vi "Set Waveform.vi"(7 "Treatment of Infinity/NaN":T1, 8 "error in (no error)":errorcluster, 10 "waveform":waveform(dbl), 11 "JSON Object in":refnum<class "JSON Object.lvclass">) -> (0 "error out":errorcluster, 3 "JSON Object out":refnum<class "JSON Object.lvclass">)   [LabVIEW 2020, in "Library Commun.lvlib" / "JSON Object.lvclass"]
uses:
  JSON Object.lvclass
  C:/Users/ngarcin/OneDrive - Altyor/Standard TB/Class/JSON API/JSON Value/JSON Value.lvclass
  JSON Scalar/Infinity&NaN.ctl
  JSON Array/JSON Array.lvclass
  JSON Scalar/JSON Scalar.lvclass
  Variant JSON/Variant JSON.lvlib
  support/JSON support.lvlib
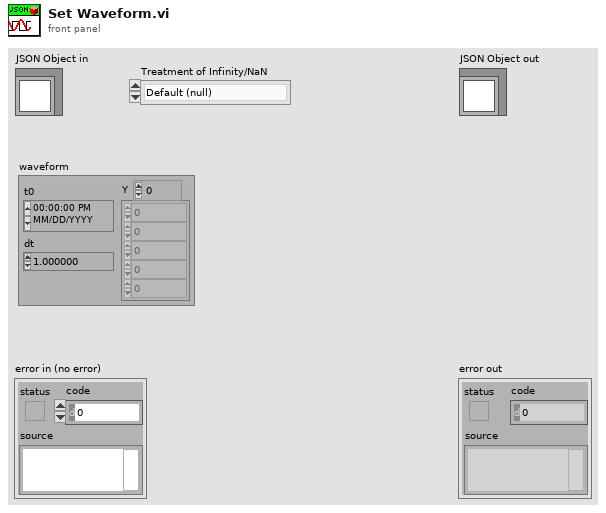
[diagram p1: front panel]
types:
  T1 = typedef "Library Commun.lvlib/JSON support.lvlib/Infinity&NaN.ctl" = enum16{"Default (null)", "Extended", "LabVIEW extensions"}
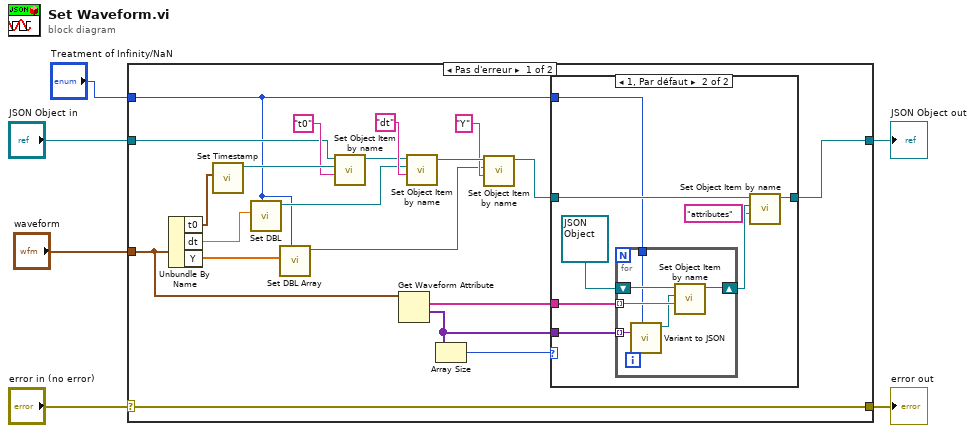
[diagram p0: block diagram]
diagram:
  n1 = case shown="Pas d'erreur" "error in (no error)" {
    selector: "error in (no error)" -> [w26 w43]
    tunnel: [w26 w43] -> w5
    tunnel: [w8 w42] -> w3
    tunnel: "JSON Object in" -> [w9 w42]
    tunnel: "waveform" -> [w25 _]
    tunnel: "Treatment of Infinity/NaN" -> [w7 _]
    frame No Error {
      n2 = Unbundle By Name(w25) -> ("t0"=w23:timestamp, "dt"=w24:dbl, "Y"=w22:dbl[])
      n3 = call "Set Timestamp.vi"("Time Stamp"=w23) -> ("JSON Scalar out"=w20:refnum<class "JSON Scalar.lvclass">)  [unwired: 9 in, 1 out]
      n4 = call "Set DBL.vi"("Treatment of Infinity/NaN"=w7, "Numeric"=w24) -> ("JSON Scalar out"=w16:refnum<class "JSON Scalar.lvclass">)  [unwired: 8 in, 1 out]
      n5 = call "Set DBL Array.vi"("Treatment of Infinity/NaN"=w7, "Array of numbers"=w22) -> ("JSON Array out"=w13:refnum<class "JSON Array.lvclass">)  [unwired: 8 in, 1 out]
      n6 = call "Set Object Item by name.vi"("name"="t0", "Value"=w20, "JSON Object in"=w9) -> ("JSON Object out"=w17:refnum<class "JSON Object.lvclass">)  [unwired: 6 in, 2 out]
      n7 = Get Waveform Attribute(7:w25) -> (1:w11:variant[], 2:w12:string[])  [unwired: 3 in, 2 out]
      n8 = call "Set Object Item by name.vi"("name"="dt", "Value"=w16, "JSON Object in"=w17) -> ("JSON Object out"=w15:refnum<class "JSON Object.lvclass">)  [unwired: 6 in, 2 out]
      n9 = Array Size(array=w11) -> (size(s)=w21:i32)
      n10 = call "Set Object Item by name.vi"("name"="Y", "Value"=w13, "JSON Object in"=w15) -> ("JSON Object out"=w10:refnum<class "JSON Object.lvclass">)  [unwired: 6 in, 2 out]
      n11 = case shown="1, Par défaut" w21 {
        tunnel: w12 -> [_ w35]
        tunnel: w11 -> [_ w34]
        tunnel: w10 -> [w27 w33]
        tunnel: [w27 w29] -> w8
        tunnel: w7 -> [_ w28]
        frame 0 {
        }
        frame 1, Default {
          n12 = for {
            tunnel: w35 -> [w41] mode=indexing
            tunnel: w34 -> [w40] mode=indexing
            shift-right: [w37] -> w31
            shift-left: refnum<class "JSON Object.lvclass"> refnum ("JSON Object in") -> [w38]
            tunnel: w28 -> [w36]
            n13 = call "Variant to JSON.vi"("Treatment of Infinity/NaN"=w36, "Variant"=w40) -> ("JSON Value out"=w39:refnum<class "JSON Value.lvclass">)  [unwired: 8 in, 1 out]
            n14 = call "Set Object Item by name.vi"("name"=w41, "Value"=w39, "JSON Object in"=w38) -> ("JSON Object out"=w37:refnum<class "JSON Object.lvclass">)  [unwired: 6 in, 2 out]
          }
          n15 = call "Set Object Item by name.vi"("name"="attributes", "Value"=w31, "JSON Object in"=w33) -> ("JSON Object out"=w29:refnum<class "JSON Object.lvclass">)  [unwired: 6 in, 2 out]
        }
      }
    }
    frame Error {
    }
  }
  "error out" <- w5
  "JSON Object out" <- w3
